vi "Read Atts.vi"(8 "error in (no error)":errorcluster, 11 "network in":refnum<class "network.lvclass">) -> (0 "error out":errorcluster, 1 "IF_Band":dbl, 2 "Stop":dbl, 3 "network out":refnum<class "network.lvclass">, 4 "Points":i32, 5 "Start":dbl)   [LabVIEW 2015, in "network.lvclass"]
uses:
  network.lvclass
  network.lvclass/network.ctl
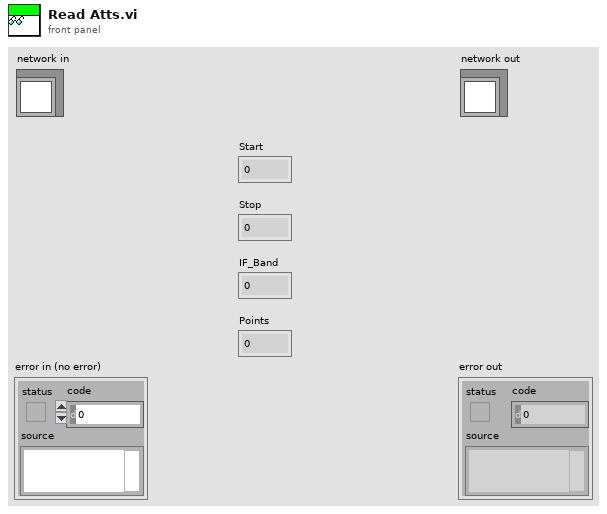
[diagram p1: front panel]
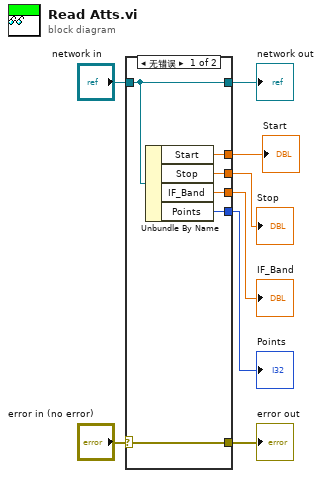
[diagram p0: block diagram]
diagram:
  n1 = case shown="无错误" "error in (no error)" {
    selector: "error in (no error)" -> [w14 w15]
    tunnel: [w14 w15] -> w7
    tunnel: [w13 w16] -> w5
    tunnel: "network in" -> [w13 w16]
    tunnel: [w12 _] -> w4
    tunnel: [w11 _] -> w3
    tunnel: [w10 _] -> w2
    tunnel: [w9 _] -> w1
    frame No Error {
      n2 = Unbundle By Name(w13) -> ("Start"=w12:dbl, "Stop"=w11:dbl, "IF_Band"=w10:dbl, "Points"=w9:i32)
    }
    frame Error {
    }
  }
  "error out" <- w7
  "network out" <- w5
  "Stop" <- w3
  "IF_Band" <- w2
  "Points" <- w1
  "Start" <- w4
